vi "frw_csv_edf_paths.vi"(6 "eeg_device":T1, 9 "file_extension":string, 10 "filename":string, 11 "directory path":path) -> (2 "path edf":path, 3 "path csv":path)   [LabVIEW 2013]
uses:
  gui/type_def/device.ctl
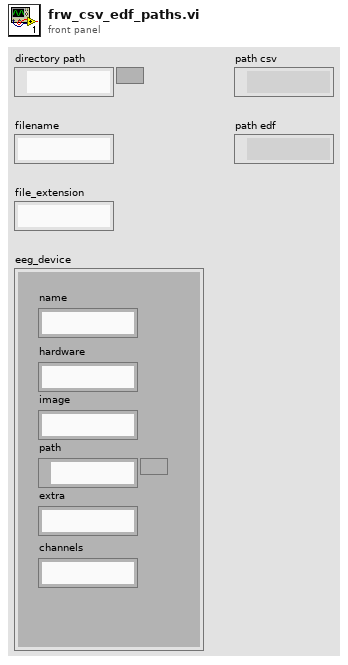
[diagram p1: front panel]
types:
  T1 = typedef "device.ctl" = cluster{"name":string, "hardware":string, "image":string, "path":path, "extra":string, "channels":string}
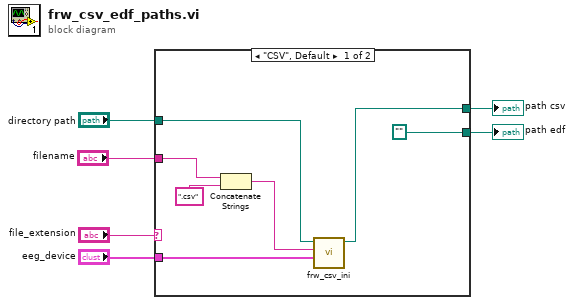
[diagram p0: block diagram]
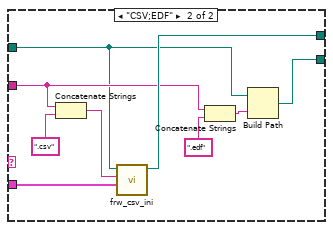
[diagram p2: hidden frame]
diagram:
  n1 = case shown="\"CSV\", Default" "file_extension" {
    tunnel: "directory path" -> [w11 w15]
    tunnel: "eeg_device" -> [w9 w22]
    tunnel: "filename" -> [w10 w17]
    tunnel: [w8 w19] -> w4
    tunnel: [path "" w14] -> w5
    frame "CSV", Default {
      n2 = Concatenate Strings(w10, ".csv" ("string")) -> (w12:string)
      n3 = call "frw_csv_ini.vi"("eeg_device"=w9, "file_name"=w12, "folder"=w11) -> ("path out"=w8:path)  [unwired: 7 in, 1 out]
    }
    frame "CSV;EDF" {
      n4 = Concatenate Strings(w17, ".csv" ("string")) -> (w20:string)
      n5 = call "frw_csv_ini.vi"("eeg_device"=w22, "file_name"=w20, "folder"=w15) -> ("path out"=w19:path)  [unwired: 7 in, 1 out]
      n6 = Concatenate Strings(w17, ".edf" ("string")) -> (w16:string)
      n7 = Build Path(base path=w15, name or relative path=w16) -> (appended path=w14:path)
    }
  }
  "path edf" <- w5
  "path csv" <- w4
